vi "Read Global Stop.vi"(11 "Template in":refnum<class "Template.lvclass">) -> (2 "Global Stop Event":refnum<user-event>, 3 "Global Stop Notifier":refnum<notifier>)   [LabVIEW 2020, in "Template.lvlib" / "Template.lvclass"]
uses:
  Template.lvclass
  Template.lvclass/Template.ctl
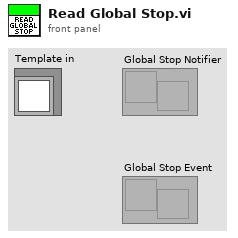
[diagram p1: front panel]
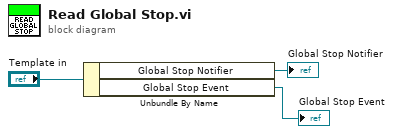
[diagram p0: block diagram]
diagram:
  n1 = Unbundle By Name("Template in") -> ("Global Stop Notifier"=→"Global Stop Notifier":refnum<notifier>, "Global Stop Event"=→"Global Stop Event":refnum<user-event>)
